vi "Create Top Level.vi"(9 "Alias":string, 10 "Actor":refnum<class "Actor.lvclass">) -> ()   [LabVIEW 2021, in "jettl.lvlib" / "jettl.lvclass"]
uses:
  jettl.lvclass
  Actor/Actor/Actor.lvclass
  jettl.lvclass/jettl.ctl
  jettl.lvlib
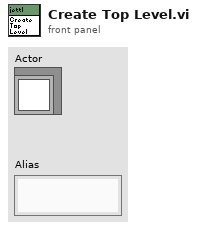
[diagram p1: front panel]
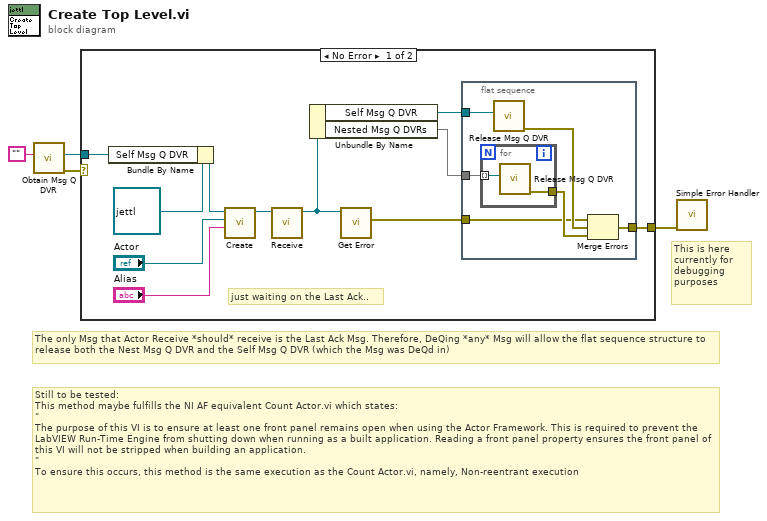
[diagram p0: block diagram]
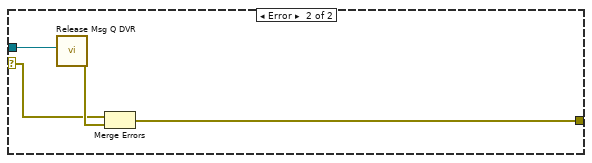
[diagram p2: hidden frame]
diagram:
  # "Still to be tested:\nThis method maybe fulfills the NI AF equivalent Count Actor.vi which states:\n\"\nThe purpose of this VI is to ensure at least one front panel remains open when using the Actor Framework. This is required to prevent the LabVIEW Run-Time Engine from shutting down when running as a built application. Reading a front panel property ensures the front panel of this VI will not be stripped when building an application.\n\"\nTo ensure this occurs, this method is the same execution as the Count Actor.vi, namely, Non-reentrant execution"
  # "This is here currently for debugging purposes"
  # "The only Msg that Actor Receive *should* receive is the Last Ack Msg. Therefore, DeQing *any* Msg will allow the flat sequence structure to release both the Nest Msg Q DVR and the Self Msg Q DVR (which the Msg was DeQd in)"
  n1 = call "Obtain Msg Q DVR.vi"("Msg Q DVR Alias"="") -> ("error out"=w1:errorcluster, "Msg Q DVR"=w4:refnum<data-value>)  [unwired: 9 in]
  n2 = case shown="No Error" w1 {
    selector: w1 -> [_ w24]
    tunnel: w4 -> [w14 w27]
    tunnel: [w13 w26] -> w3
    frame No Error {
      # "just waiting on the Last Ack.."
      n3 = Bundle By Name(cluster=refnum<class "jettl.lvclass"> refnum ("Self Actor in"), "Self Msg Q DVR"=w14) -> (w11:refnum<class "jettl.lvclass">)
      n4 = call-dynamic "Create.vi"("Alias"="Alias", "Actor"="Actor", "jettl in"=w11) -> ("jettl out"=w7:refnum<class "jettl.lvclass">)  [unwired: 8 in]
      n5 = call-dynamic "Receive.vi"("jettl in"=w7) -> ("jettl out"=w5:refnum<class "jettl.lvclass">)  [unwired: 9 in, 1 out]
      n6 = Unbundle By Name(w5) -> ("Self Msg Q DVR"=w15:refnum<data-value>, "Nested Msg Q DVRs"=w12:set{refnum<data-value>})
      n7 = call-dynamic "Get Error.vi"("jettl in"=w5) -> ("Error"=w6:errorcluster)  [unwired: 10 in]
      n8 = flat-sequence {
        tunnel: w15 -> [w21]
        tunnel: [w20] -> w13
        tunnel: w12 -> [w19]
        tunnel: w6 -> [w16]
        frame #0 {
          n9 = for {
            tunnel: w19 -> [w23] mode=indexing
            tunnel: [w22] -> w18
            n10 = call "Release Msg Q DVR.vi"("Msg Q DVR"=w23) -> ("error out"=w22:errorcluster)  [unwired: 10 in]
          }
          n11 = call "Release Msg Q DVR.vi"("Msg Q DVR"=w21) -> ("error out"=w17:errorcluster)  [unwired: 10 in]
          n12 = Merge Errors(w16, w17, w18) -> (w20:errorcluster)
        }
      }
    }
    frame Error {
      n13 = call "Release Msg Q DVR.vi"("Msg Q DVR"=w27) -> ("error out"=w25:errorcluster)  [unwired: 10 in]
      n14 = Merge Errors(w24, w25) -> (w26:errorcluster)
    }
  }
  n15 = call <vilib>:"Simple Error Handler.vi"("error in (no error)"=w3) -> ()  [unwired: 4 in, 5 out]
